vi "PH_PSDBWriter.set PSDB Dataset.vi"(0 "VI in":refnum<vi>, 2 "PSDB Dataset":T1, 5 "error in (no error)":errorcluster) -> (14 "VI out":refnum<vi>, 19 "error out":errorcluster)   [LabVIEW 2014, in "PH_PSDBWriter.lvlib"]
doc: "This VI sets the PSDB Dataset to own attributes."
uses:
  PH_PSDBWriter.lvlib
  PH_PSDBWriter.PSDB Dataset.ctl
  PH_PSDBWriter.2D dataset.ctl
  CSlibraries-extern/psdb_lv/PSDB_AxisDescription.ctl
  PH_PSDBWriter.Boolean dataset.ctl
  PH_PSDBWriter.Image dataset.ctl
  <vilib>/vision/Image Controls.llb/IMAQ Image.ctl
  PH_PSDBWriter.Numeric dataset.ctl
  PH_PSDBWriter.String dataset.ctl
  CSlibraries-extern/psdb_lv/PSDB.lvlib
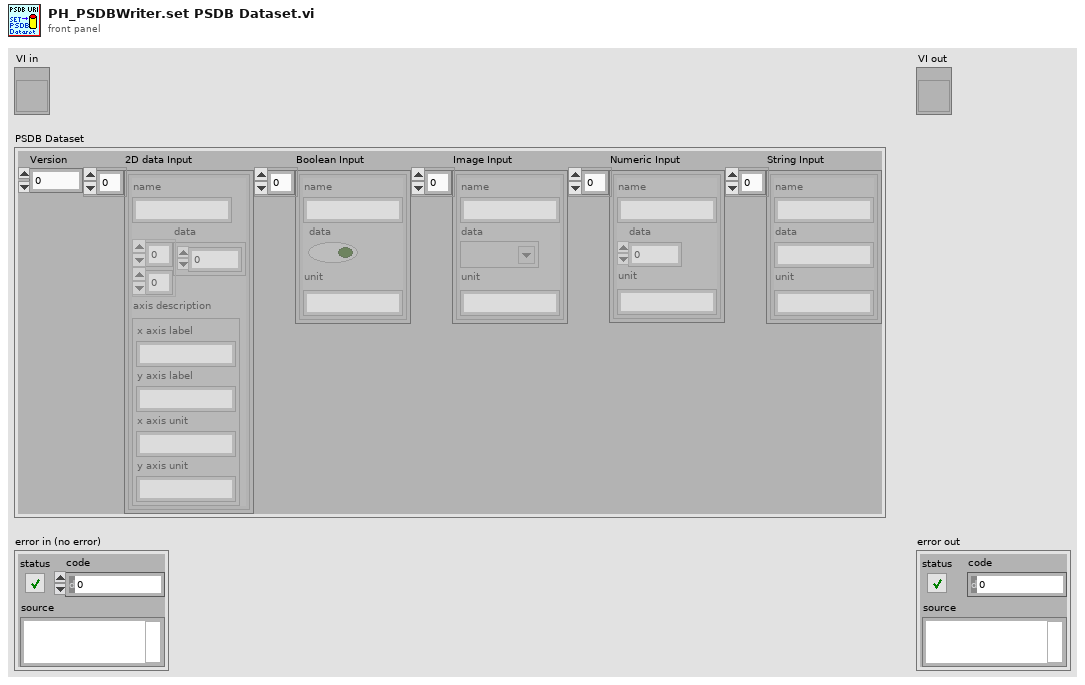
[diagram p1: front panel]
types:
  T1 = typedef "PH_PSDBWriter.lvlib/PH_PSDBWriter.PSDB Dataset.ctl" = cluster{"Version":i32, "2D data Input":T2[], "Boolean Input":T4[], "Image Input":T5[], "Numeric Input":T7[], "String Input":T8[]}
  T2 = typedef "PH_PSDBWriter.lvlib/PH_PSDBWriter.2D dataset.ctl" = cluster{"name":string, "data":dbl[][], "axis description":T3}
  T3 = typedef "PSDB.lvlib/PSDB_AxisDescription.ctl" = cluster{"x axis label":string, "y axis label":string, "x axis unit":string, "y axis unit":string}
  T4 = typedef "PH_PSDBWriter.lvlib/PH_PSDBWriter.Boolean dataset.ctl" = cluster{"name":string, "data":bool, "unit":string}
  T5 = typedef "PH_PSDBWriter.lvlib/PH_PSDBWriter.Image dataset.ctl" = cluster{"name":string, "data":T6, "unit":string}
  T6 = typedef "IMAQ Image.ctl" = refnum<image>
  T7 = typedef "PH_PSDBWriter.lvlib/PH_PSDBWriter.Numeric dataset.ctl" = cluster{"name":string, "data":dbl, "unit":string}
  T8 = typedef "PH_PSDBWriter.lvlib/PH_PSDBWriter.String dataset.ctl" = cluster{"name":string, "data":string, "unit":string}
  T9 = typedef "PH_PSDBWriter.lvlib/PH_PSDBWriter.i attribute.ctl" = cluster{"PSDB Status Service ID":i32, "Instance ID":i32, "Shot #":i32, "Subsystem":T10, "Data Status":T11, "Ref PSDB Status":refnum<vi>, "PSDB Error Code":i32, "PSDB Dataset":T1, "PSDB Thread":cluster{"Ref":refnum<vi>, "Q-Ref":refnum<queue>}, "PSDB Credentials":T12}
  T10 = typedef "PH_PSDBWriter.lvlib/PH_PSDBWriter.PHELIX-Subsystems.ctl" = i32
  T11 = typedef "PH_PSDBWriter.lvlib/PH_PSDBWriter.Data Status.ctl" = i16
  T12 = typedef "PH_Common.lvlib/PH_Connection.PSDB Credentials.ctl" = cluster{"PW":string, "ID":string, "DS":string}
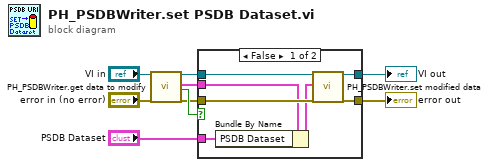
[diagram p0: block diagram]
diagram:
  n1 = call "PH_PSDBWriter.get data to modify.vi"("i ref in"="VI in", "error in (no error)"="error in (no error)") -> ("i ref out"=w5:refnum<vi>, "i attribute"=w7:T9, "timed out"=w8:bool, "error out"=w2:errorcluster)  [unwired: 14 in]
  n2 = case shown="False" w8 {
    tunnel: w2 -> [w16 w17]
    tunnel: [w15 w17] -> w3
    tunnel: w5 -> [w14 w18]
    tunnel: [w13 w18] -> w6
    tunnel: w7 -> [w12 _]
    tunnel: "PSDB Dataset" -> [w10 _]
    frame False {
      n3 = Bundle By Name(cluster=w12, "PSDB Dataset"=w10) -> (w11:T9)
      n4 = call "PH_PSDBWriter.set modified data.vi"("i ref in"=w14, "i attribute"=w11, "error in (no error)"=w16) -> ("i ref out"=w13:refnum<vi>, "error out"=w15:errorcluster)  [unwired: 15 in]
    }
    frame True {
    }
  }
  "VI out" <- w6
  "error out" <- w3
